vi "CreateTable.vi"() -> ()   [LabVIEW 2020]
uses:
  <vilib>/addons/database/Auxilliary.llb/DB Tools Column Info.ctl
  <vilib>/addons/database/Auxilliary.llb/DB Tools DataTypes.ctl
  <vilib>/addons/database/NI_Database_API.lvlib
panel:
  in  "error in (no error)":errorcluster
  out "error out":errorcluster
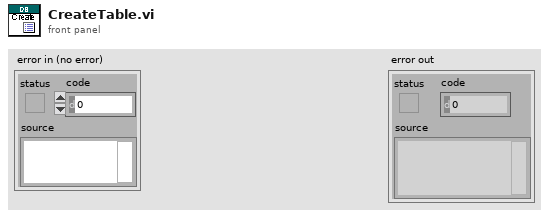
[diagram p1: front panel]
types:
  T1 = typedef "NI_Database_API.lvlib/DB Tools Column Info.ctl" = cluster{"column name":string, "data type":T2, "size":i32, "allow null?":bool}
  T2 = typedef "NI_Database_API.lvlib/DB Tools DataTypes.ctl" = enum16{"String", "Long (I32)", "Single (SGL)", "Double (DBL)", "Date/Time", "Binary"}
  T3 = typedef "NI_Database_API.lvlib/Conn ObjectReference.ctl" = refnum<k1>
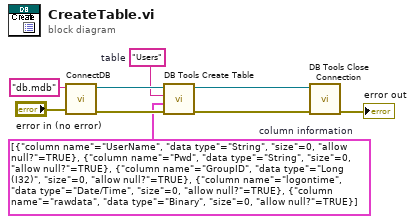
[diagram p0: block diagram]
diagram:
  w1 = T1[] [{"column name"="UserName", "data type"=enum."String", "size"=0, "allow null?"=TRUE}, {"column name"="Pwd", "data type"=enum."String", "size"=0, "allow null?"=TRUE}, {"column name"="GroupID", "data type"=enum."Long (I32)", "size"=0, "allow null?"=TRUE}, {"column name"="logontime", "data type"=enum."Date/Time", "size"=0, "allow null?"=TRUE}, {"column name"="rawdata", "data type"=enum."Binary", "size"=0, "allow null?"=TRUE}]  # column information
  w2 = "Users"  # table
  n1 = call "ConnectDB.vi"("error in (no error)"="error in (no error)", "Filename"="db.mdb") -> ("error out"=w7:errorcluster, "DB Conn"=w8:T3)  [unwired: 8 in]
  n2 = call <vilib>:"DB Tools Create Table.vi"("error in (no error)"=w7, "column information"=w1, "table"=w2, "connection reference"=w8) -> ("error out"=w6:errorcluster, "connection reference out"=w5:T3)  [unwired: 4 in]
  n3 = call <vilib>:"DB Tools Close Connection.vi"("error in (no error)"=w6, "connection reference"=w5) -> ("error out"=→"error out":errorcluster)  [unwired: 5 in]
